vi "PLC Primitive Byte Stream to Data String.vi"(8 "error in (no error)":errorcluster, 9 "PLC Type":T1, 10 "Byte Stream":u8[](array[numeric]), 11 "TwinCAT ADS in":refnum<class "TwinCAT ADS.lvclass">) -> (0 "error out":errorcluster, 1 "Data String":string, 2 "Type Descriptor":i16[](array[numeric]), 3 "TwinCAT ADS out":refnum<class "TwinCAT ADS.lvclass">)   [LabVIEW 2018, in "TwinCAT ADS.lvclass"]
uses:
  TwinCAT ADS.lvclass
  Controls/PLC Type.ctl
  dd5e40b3-f89d-44d0-b911-1f2dc1f1e391.vi
  9a8c356b-cf55-4838-9201-0532b80217b2.vi
  06482052-d1f9-4f29-aca9-908031c6a69f.vi
  b9242781-96b0-446e-9150-452b1084ed54.vi
  5fbe6976-0b86-40a2-b7b6-3748894f0071.vi
  c4de1741-fffd-4fed-ba25-d7b4acbf0555.vi
  20356124-05d2-4a04-a5d1-e69adc4c58c2.vi
  67ddb754-0fbe-43d9-9e61-34d6659124ef.vi
  e3d41cb3-d20e-45e9-8252-e41884a8f4d0.vi
  46ba2a54-cc07-4222-9a0e-bd972edfcef0.vi
  6b416cf7-30dc-48a3-9278-9d800f443678.vi
  5857d013-9824-4299-a2d7-53efdc0d26c5.vi
  006b0e7e-7e80-41f3-be4e-1f3da8479fae.vi
  28d9c90b-5f2a-4c58-95e2-5fc46303b0fd.vi
  99b7bc4a-962e-4818-aa5d-444f23f83b11.vi
  8b7c42c8-9170-4542-8f35-15cbeddc22cb.vi
  65a091fa-0bd2-4a35-ae2b-3fa5e90d1994.vi
  4b7d3a7d-7f1b-46f0-9357-48cb72148c56.vi
  b431183c-2ad5-4c6d-9bfa-a53b18913682.vi
  30c6c28a-53c3-4e33-80b1-b22f521e1f67.vi
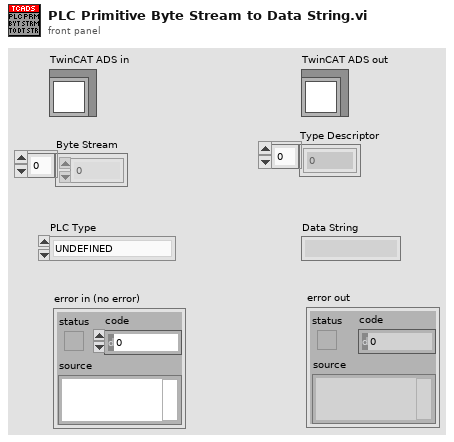
[diagram p1: front panel]
types:
  T1 = typedef "TwinCAT ADS.lvclass/PLC Type.ctl" = enum16{"UNDEFINED", "INT", "DINT", "REAL", "LREAL", "SINT", "BYTE", "UINT", "UDINT", "LINT", "ULINT", "STRING", "WSTRING", "BOOL", "TIME", "LTIME", "DATE", "DT", "TOD", "ARRAY", "JAGGED ARRAY", "STRUCT", "FUNCTION BLOCK", "UNION", "POINTER", "USER DEFINED"}
  T2 = typedef "LVDateTimeRec.ctl" = cluster{"fractional second":dbl, "second":i32, "minute":i32, "hour":i32, "day of month":i32, "month":i32, "year":i32, "day of week":i32, "day of year":i32, "DST":i32}
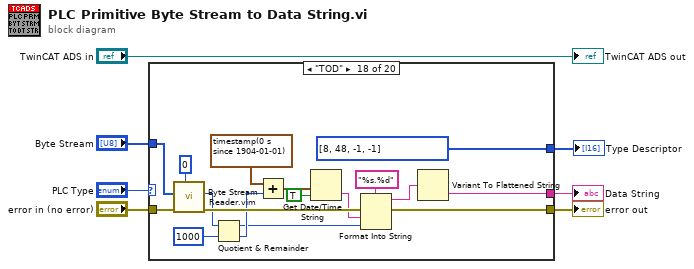
[diagram p0: block diagram]
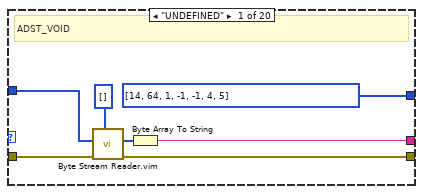
[diagram p2: hidden frame]
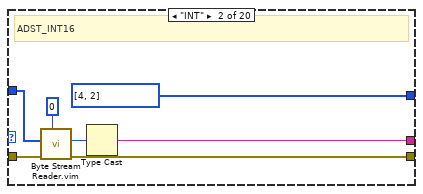
[diagram p3: hidden frame]
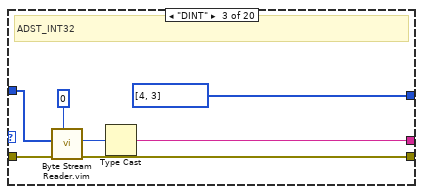
[diagram p4: hidden frame]
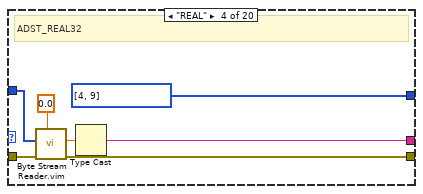
[diagram p5: hidden frame]
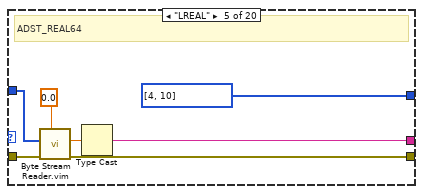
[diagram p6: hidden frame]
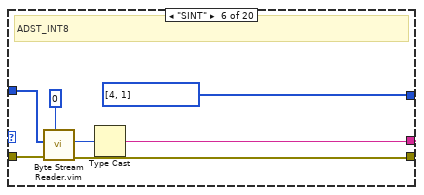
[diagram p7: hidden frame]
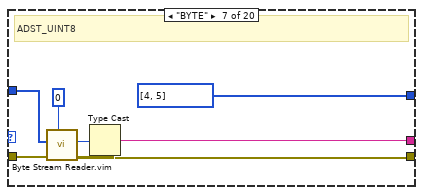
[diagram p8: hidden frame]
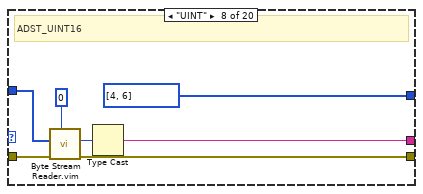
[diagram p9: hidden frame]
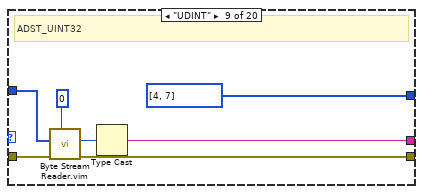
[diagram p10: hidden frame]
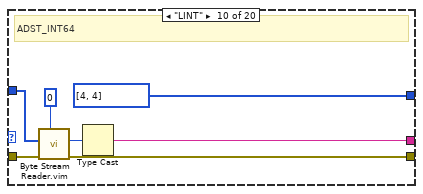
[diagram p11: hidden frame]
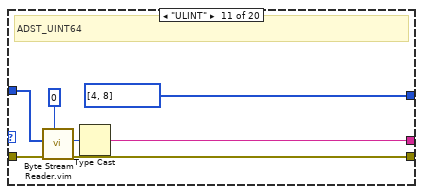
[diagram p12: hidden frame]
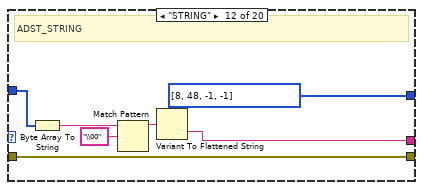
[diagram p13: hidden frame]
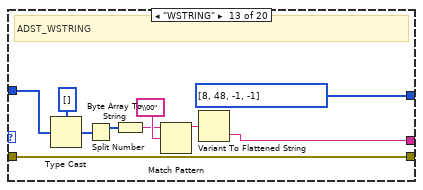
[diagram p14: hidden frame]
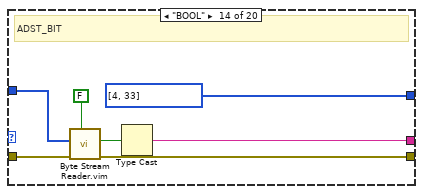
[diagram p15: hidden frame]
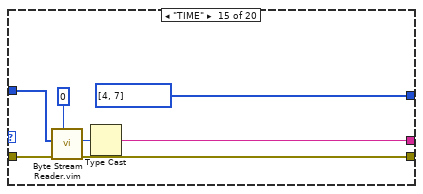
[diagram p16: hidden frame]
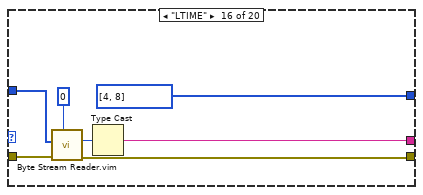
[diagram p17: hidden frame]
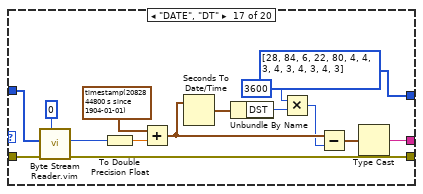
[diagram p18: hidden frame]
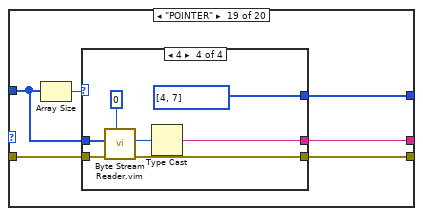
[diagram p19: hidden frame]
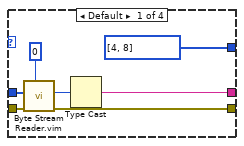
[diagram p20: hidden frame]
diagram:
  n1 = case shown="\"TOD\"" "PLC Type" {
    tunnel: [w9 w17 w23 w30 w37 w44 w51 w58 w65 w72 w79 w87 w94 w103 w111 w117 w124 w138 w157 w190] -> w5
    tunnel: "error in (no error)" -> [w14 w21 w28 w35 w42 w49 w56 w63 w70 w77 w84 w88 w95 w108 w115 w122 w136 w153 w160 w192]
    tunnel: [w11 w20 w27 w34 w41 w48 w55 w62 w68 w75 w82 w88 w95 w106 w113 w120 w133 w144 w156 w192] -> w4
    tunnel: "Byte Stream" -> [w13 w19 w26 w33 w40 w47 w54 w61 w69 w76 w83 w91 w100 w107 w114 w121 w135 w151 w158 w191]
    tunnel: [i16[] [14, 64, 1, -1, -1, 4, 5] ("Type Descriptor") i16[] [4, 2] ("Type Descriptor") i16[] [4, 3] ("Type Descriptor") i16[] [4, 9] ("Type Descriptor") i16[] [4, 10] ("Type Descriptor") i16[] [4, 1] ("Type Descriptor") i16[] [4, 5] ("Type Descriptor") i16[] [4, 6] ("Type Descriptor") i16[] [4, 7] ("Type Descriptor") i16[] [4, 4] ("Type Descriptor") i16[] [4, 8] ("Type Descriptor") i16[] [8, 48, -1, -1] ("Type Descriptor") i16[] [8, 48, -1, -1] ("Type Descriptor") i16[] [4, 33] ("Type Descriptor") i16[] [4, 7] ("Type Descriptor") i16[] [4, 8] ("Type Descriptor") i16[] [28, 84, 6, 22, 80, 4, 4, 3, 4, 3, 4, 3, 4, 3] ("Type Descriptor") i16[] [8, 48, -1, -1] ("Type Descriptor") w155 i16[] [14, 64, 1, -1, -1, 4, 5] ("Type Descriptor")] -> w1
    frame "UNDEFINED" {
      # "ADST_VOID"
      n2 = call "Byte Stream Reader.vim"("Type"=u8[] [], "error in (no error)"=w14, "Byte Stream"=w13) -> ("error out"=w11:errorcluster, "Value"=w10:u8[])  [unwired: 7 in]
      n3 = Byte Array To String(unsigned byte array=w10) -> (string=w9:string)
    }
    frame "INT" {
      # "ADST_INT16"
      n4 = call "Byte Stream Reader.vim"("Type"=i16 0, "error in (no error)"=w21, "Byte Stream"=w19) -> ("error out"=w20:errorcluster, "Value"=w18:i16)  [unwired: 7 in]
      n5 = Type Cast(x=w18) -> (*(type *) &x=w17:string)  [unwired: 1 in]
    }
    frame "DINT" {
      # "ADST_INT32"
      n6 = call "Byte Stream Reader.vim"("Type"=0, "error in (no error)"=w28, "Byte Stream"=w26) -> ("error out"=w27:errorcluster, "Value"=w25:i32)  [unwired: 7 in]
      n7 = Type Cast(x=w25) -> (*(type *) &x=w23:string)  [unwired: 1 in]
    }
    frame "REAL" {
      # "ADST_REAL32"
      n8 = call "Byte Stream Reader.vim"("Type"=sgl 0.0, "error in (no error)"=w35, "Byte Stream"=w33) -> ("error out"=w34:errorcluster, "Value"=w32:sgl)  [unwired: 7 in]
      n9 = Type Cast(x=w32) -> (*(type *) &x=w30:string)  [unwired: 1 in]
    }
    frame "LREAL" {
      # "ADST_REAL64"
      n10 = call "Byte Stream Reader.vim"("Type"=0.0, "error in (no error)"=w42, "Byte Stream"=w40) -> ("error out"=w41:errorcluster, "Value"=w39:dbl)  [unwired: 7 in]
      n11 = Type Cast(x=w39) -> (*(type *) &x=w37:string)  [unwired: 1 in]
    }
    frame "SINT" {
      # "ADST_INT8"
      n12 = call "Byte Stream Reader.vim"("Type"=i8 0, "error in (no error)"=w49, "Byte Stream"=w47) -> ("error out"=w48:errorcluster, "Value"=w46:i8)  [unwired: 7 in]
      n13 = Type Cast(x=w46) -> (*(type *) &x=w44:string)  [unwired: 1 in]
    }
    frame "BYTE" {
      # "ADST_UINT8"
      n14 = call "Byte Stream Reader.vim"("Type"=u8 0, "error in (no error)"=w56, "Byte Stream"=w54) -> ("error out"=w55:errorcluster, "Value"=w53:u8)  [unwired: 7 in]
      n15 = Type Cast(x=w53) -> (*(type *) &x=w51:string)  [unwired: 1 in]
    }
    frame "UINT" {
      # "ADST_UINT16"
      n16 = call "Byte Stream Reader.vim"("Type"=u16 0, "error in (no error)"=w63, "Byte Stream"=w61) -> ("error out"=w62:errorcluster, "Value"=w60:u16)  [unwired: 7 in]
      n17 = Type Cast(x=w60) -> (*(type *) &x=w58:string)  [unwired: 1 in]
    }
    frame "UDINT" {
      # "ADST_UINT32"
      n18 = call "Byte Stream Reader.vim"("Type"=u32 0, "error in (no error)"=w70, "Byte Stream"=w69) -> ("error out"=w68:errorcluster, "Value"=w67:u32)  [unwired: 7 in]
      n19 = Type Cast(x=w67) -> (*(type *) &x=w65:string)  [unwired: 1 in]
    }
    frame "LINT" {
      # "ADST_INT64"
      n20 = call "Byte Stream Reader.vim"("Type"=i64 0, "error in (no error)"=w77, "Byte Stream"=w76) -> ("error out"=w75:errorcluster, "Value"=w74:i64)  [unwired: 7 in]
      n21 = Type Cast(x=w74) -> (*(type *) &x=w72:string)  [unwired: 1 in]
    }
    frame "ULINT" {
      # "ADST_UINT64"
      n22 = call "Byte Stream Reader.vim"("Type"=u64 0, "error in (no error)"=w84, "Byte Stream"=w83) -> ("error out"=w82:errorcluster, "Value"=w80:u64)  [unwired: 7 in]
      n23 = Type Cast(x=w80) -> (*(type *) &x=w79:string)  [unwired: 1 in]
    }
    frame "STRING" {
      # "ADST_STRING"
      n24 = Byte Array To String(unsigned byte array=w91) -> (string=w90:string)
      n25 = Match Pattern(string=w90, regular expression="\\00") -> (before substring=w86:string)  [unwired: 1 in, 3 out]
      n26 = Variant To Flattened String(Variant=w86) -> (data string=w87:string)  [unwired: 1 out]
    }
    frame "WSTRING" {
      # "ADST_WSTRING"
      n27 = Type Cast(type=u16[] [] ("Byte Stream"), x=w100) -> (*(type *) &x=w96:u16[])
      n28 = Split Number(x=w96) -> (hi(x)=w97:u8[])  [unwired: 1 out]
      n29 = Byte Array To String(unsigned byte array=w97) -> (string=w98:string)
      n30 = Match Pattern(string=w98, regular expression="\\00") -> (before substring=w92:string)  [unwired: 1 in, 3 out]
      n31 = Variant To Flattened String(Variant=w92) -> (data string=w94:string)  [unwired: 1 out]
    }
    frame "BOOL" {
      # "ADST_BIT"
      n32 = call "Byte Stream Reader.vim"("Type"=FALSE, "error in (no error)"=w108, "Byte Stream"=w107) -> ("error out"=w106:errorcluster, "Value"=w105:bool)  [unwired: 7 in]
      n33 = Type Cast(x=w105) -> (*(type *) &x=w103:string)  [unwired: 1 in]
    }
    frame "TIME" {
      n34 = call "Byte Stream Reader.vim"("Type"=u32 0, "error in (no error)"=w115, "Byte Stream"=w114) -> ("error out"=w113:errorcluster, "Value"=w112:u32)  [unwired: 7 in]
      n35 = Type Cast(x=w112) -> (*(type *) &x=w111:string)  [unwired: 1 in]
    }
    frame "LTIME" {
      n36 = call "Byte Stream Reader.vim"("Type"=u64 0, "error in (no error)"=w122, "Byte Stream"=w121) -> ("error out"=w120:errorcluster, "Value"=w119:u64)  [unwired: 7 in]
      n37 = Type Cast(x=w119) -> (*(type *) &x=w117:string)  [unwired: 1 in]
    }
    frame "DATE", "DT" {
      n38 = call "Byte Stream Reader.vim"("Type"=u32 0, "error in (no error)"=w136, "Byte Stream"=w135) -> ("error out"=w133:errorcluster, "Value"=w132:u32)  [unwired: 7 in]
      n39 = To Double Precision Float(number=w132) -> (double precision float=w134:dbl)
      n40 = Add(x=timestamp(2082844800 s since 1904-01-01) ("time stamp"), y=w134) -> (x+y=w130:timestamp)
      n41 = Seconds To Date/Time(time stamp (now)=w130) -> (date time rec=w129:T2)  [unwired: 1 in]
      n42 = Unbundle By Name(w129) -> ("DST"=w128:i32)
      n43 = Multiply(x=3600, y=w128) -> (x*y=w126:i32)
      n44 = Subtract(x=w130, y=w126) -> (x-y=w125:timestamp)
      n45 = Type Cast(x=w125) -> (*(type *) &x=w124:string)  [unwired: 1 in]
    }
    frame "TOD" {
      n46 = call "Byte Stream Reader.vim"("Type"=u32 0, "error in (no error)"=w153, "Byte Stream"=w151) -> ("error out"=w154:errorcluster, "Value"=w143:u32)  [unwired: 7 in]
      n47 = Quotient & Remainder(x=w143, y=u32 1000) -> (x-y*floor(x/y)=w142:u32, floor(x/y)=w148:u32)
      n48 = Add(x=timestamp(0 s since 1904-01-01), y=w148) -> (x+y=w147:timestamp)
      n49 = Get Date/Time String(seconds (now)=w147, want seconds? (F)=TRUE) -> (time string=w141:string)  [unwired: 1 in, 1 out]
      n50 = Format Into String(format string="%s.%d", error in=w154, w141, w142) -> (resulting string=w139:string, error out=w144:errorcluster)  [unwired: 1 in]
      n51 = Variant To Flattened String(Variant=w139) -> (data string=w138:string)  [unwired: 1 out]
    }
    frame "POINTER" {
      n52 = Array Size(array=w158) -> (size(s)=w159:i32)
      n53 = case shown="4" w159 {
        tunnel: w160 -> [w166 w173 w180 w187]
        tunnel: w158 -> [w164 w171 w178 w185]
        tunnel: [w163 w170 w177 w184] -> w156
        tunnel: [w162 w169 w176 w183] -> w157
        tunnel: [i16[] [4, 8] ("Type Descriptor") i16[] [4, 8] ("Type Descriptor") i16[] [4, 6] ("Type Descriptor") i16[] [4, 7] ("Type Descriptor")] -> w155
        frame Default {
          n54 = call "Byte Stream Reader.vim"("Type"=u64 0, "error in (no error)"=w166, "Byte Stream"=w164) -> ("error out"=w163:errorcluster, "Value"=w167:u64)  [unwired: 7 in]
          n55 = Type Cast(x=w167) -> (*(type *) &x=w162:string)  [unwired: 1 in]
        }
        frame 1 {
          n56 = call "Byte Stream Reader.vim"("Type"=u64 0, "error in (no error)"=w173, "Byte Stream"=w171) -> ("error out"=w170:errorcluster, "Value"=w174:u64)  [unwired: 7 in]
          n57 = Type Cast(x=w174) -> (*(type *) &x=w169:string)  [unwired: 1 in]
        }
        frame 2 {
          n58 = call "Byte Stream Reader.vim"("Type"=u16 0, "error in (no error)"=w180, "Byte Stream"=w178) -> ("error out"=w177:errorcluster, "Value"=w181:u16)  [unwired: 7 in]
          n59 = Type Cast(x=w181) -> (*(type *) &x=w176:string)  [unwired: 1 in]
        }
        frame 4 {
          n60 = call "Byte Stream Reader.vim"("Type"=u32 0, "error in (no error)"=w187, "Byte Stream"=w185) -> ("error out"=w184:errorcluster, "Value"=w188:u32)  [unwired: 7 in]
          n61 = Type Cast(x=w188) -> (*(type *) &x=w183:string)  [unwired: 1 in]
        }
      }
    }
    frame Default {
      n62 = Byte Array To String(unsigned byte array=w191) -> (string=w190:string)
    }
  }
  "error out" <- w4
  "Data String" <- w5
  "Type Descriptor" <- w1
  "TwinCAT ADS out" <- "TwinCAT ADS in"
